vi "Push Data Logger Output Records.vi"(8 "error in":errorcluster, 10 "Data Logger Output":string, 11 "queue in":refnum<queue>) -> (0 "error out":errorcluster, 3 "queue out":refnum<queue>)   [LabVIEW 2013, in "Data Log Fetcher.lvlib"]
uses:
  Data Log Fetcher.lvlib
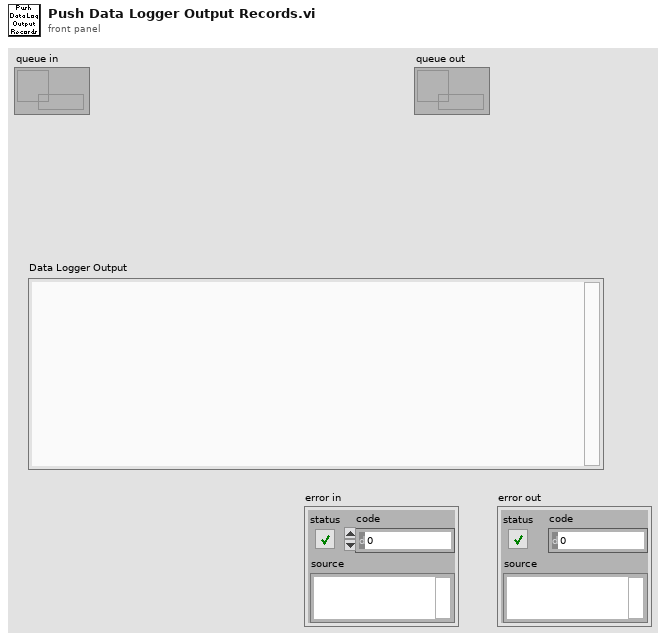
[diagram p1: front panel]
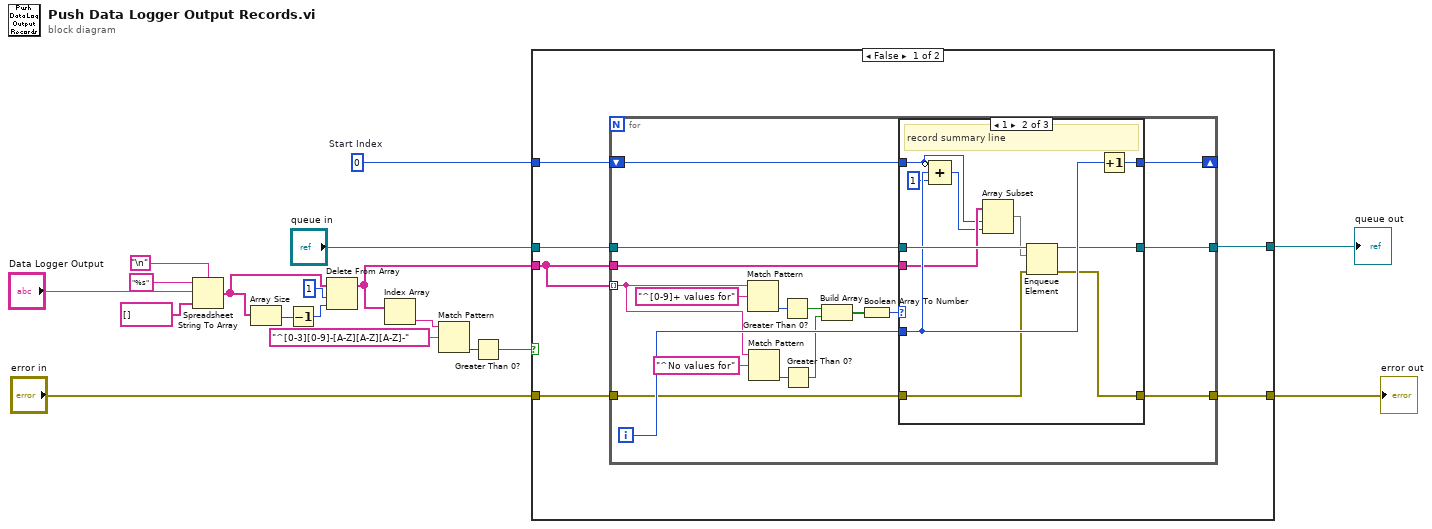
[diagram p0: block diagram]
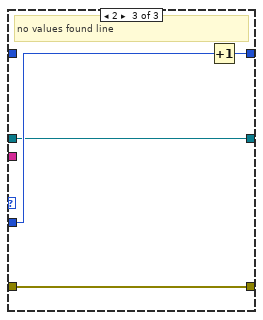
[diagram p3: hidden frame]
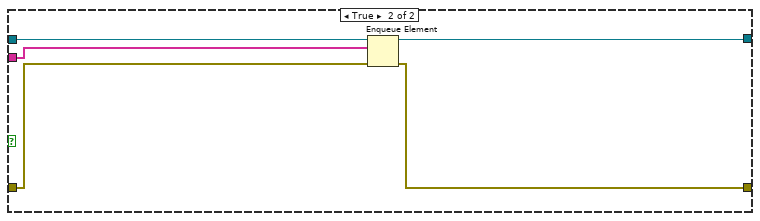
[diagram p4: hidden frame]
diagram:
  w10 = 0  # Start Index
  n1 = Spreadsheet String To Array(delimiter (Tab)="\n", format string="%s", spreadsheet string="Data Logger Output", array type (2D Dbl)=string[] []) -> (array=w16:string[])
  n2 = Array Size(array=w16) -> (size(s)=w17:i32)
  n3 = Decrement(x=w17) -> (x-1=w18:i32)
  n4 = Delete From Array(array=w16, length=1 ("index"), index=w18) -> (array with subset deleted=w3:string[])  [unwired: 1 out]
  n5 = Index Array(array=w3) -> (element=w2:string)  [unwired: 1 in]
  n6 = Match Pattern(string=w2, regular expression="^[0-3][0-9]-[A-Z][A-Z][A-Z]-") -> (offset past match=w5:i32)  [unwired: 1 in, 3 out]
  n7 = Greater Than 0?(x=w5) -> (x > 0?=w1:bool)
  n8 = case shown="False" w1 {
    tunnel: w10 -> [w24 _]
    tunnel: "queue in" -> [w23 w64]
    tunnel: "error in" -> [w22 w62]
    tunnel: [w21 w61] -> w7
    tunnel: [w20 w60] -> w6
    tunnel: w3 -> [w19 w63]
    frame False {
      n9 = for {
        tunnel: w19 -> [w26] mode=indexing
        shift-right: [w35] -> _
        shift-left: w24 -> [w36]
        tunnel: w23 -> [w39]
        tunnel: w19 -> [w37]
        tunnel: w22 -> [w28]
        tunnel: [w27] -> w21
        tunnel: [w25] -> w20
        i -> [w38]
        n10 = Match Pattern(string=w26, regular expression="^[0-9]+ values for") -> (offset past match=w40:i32)  [unwired: 1 in, 3 out]
        n11 = Match Pattern(string=w26, regular expression="^No values for") -> (offset past match=w33:i32)  [unwired: 1 in, 3 out]
        n12 = Greater Than 0?(x=w40) -> (x > 0?=w32:bool)
        n13 = Greater Than 0?(x=w33) -> (x > 0?=w31:bool)
        n14 = Build Array(w32, w31) -> (w30:bool[])
        n15 = Boolean Array To Number(Boolean array=w30) -> (number=w29:u32)
        n16 = case shown="1" w29 {
          tunnel: w39 -> [w42 w55 w56]
          tunnel: w38 -> [_ w53 w58]
          tunnel: w37 -> [_ w51 _]
          tunnel: w36 -> [w44 w49 _]
          tunnel: [w44 w54 w59] -> w35
          tunnel: w28 -> [w43 w47 w57]
          tunnel: [w43 w46 w57] -> w27
          tunnel: [w42 w45 w56] -> w25
          frame 0, Default {
          }
          frame 1 {
            # "record summary line"
            n17 = Compound Arithmetic op=ADD(invert w49, w53, 1 ("value")) -> (w50:i32)
            n18 = Array Subset(array=w51, index=w49, length=w50) -> (w48:string[])
            n19 = Enqueue Element(queue=w55, element=w48, error in (no error)=w47) -> (queue out=w45:refnum<queue>, error out=w46:errorcluster)  [unwired: 1 in, 1 out]
            n20 = Increment(x=w53) -> (x+1=w54:i32)
          }
          frame 2 {
            # "no values found line"
            n21 = Increment(x=w58) -> (x+1=w59:i32)
          }
        }
      }
    }
    frame True {
      n22 = Enqueue Element(queue=w64, element=w63, error in (no error)=w62) -> (queue out=w60:refnum<queue>, error out=w61:errorcluster)  [unwired: 1 in, 1 out]
    }
  }
  "error out" <- w7
  "queue out" <- w6
